vi "General Block Diagram.vi"() -> ()   [LabVIEW 2017]
panel:
  out "Current Forearm\nAngle":dbl
  out "Current Backarm\nAngle":dbl
  in  "Initial Parametric\nValue":dbl format="%#_13g"
  in  "Initial Forearm\nAngle":dbl format="%#_13g"
  in  "Initial Backarm\nAngle":dbl format="%#_13g"
  in  "Forearm Length":dbl format="%#_13g"
  in  "Backarm Length":dbl format="%#_13g"
  in  "New Parametric\nValue":dbl
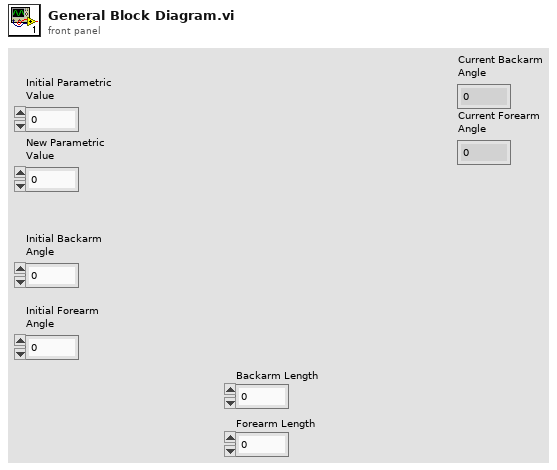
[diagram p1: front panel]
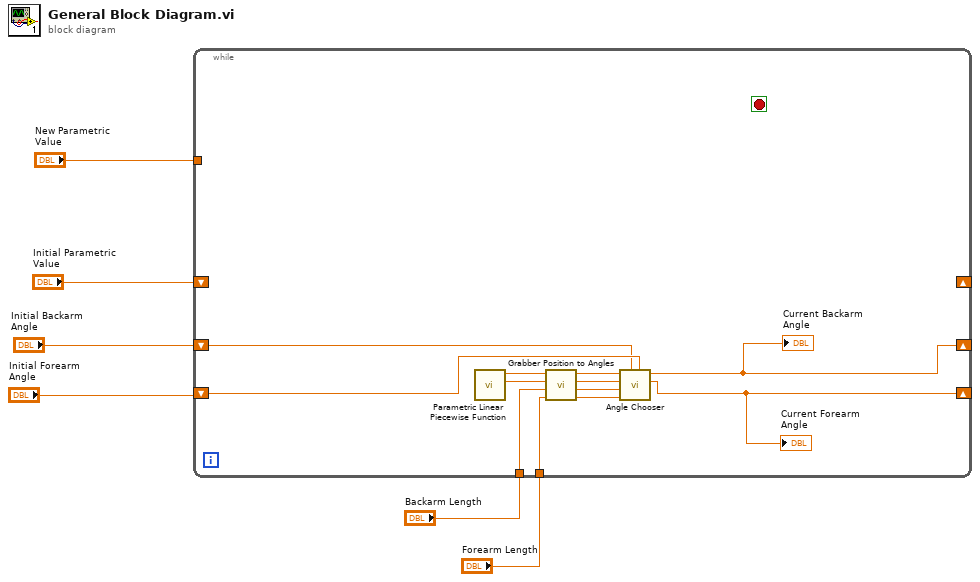
[diagram p0: block diagram]
diagram:
  n1 = while {
    shift-right: _ -> [_]
    shift-left: "Initial Parametric\nValue" -> [_]
    tunnel: "New Parametric\nValue" -> [_]
    tunnel: "Forearm Length" -> [w12]
    tunnel: "Backarm Length" -> [w11]
    shift-right: [w8] -> _
    shift-left: "Initial Backarm\nAngle" -> [w9]
    shift-right: [w7] -> _
    shift-left: "Initial Forearm\nAngle" -> [w10]
    stop <- _ stop-if-true
    n2 = call "Parametric Linear Piecewise Function.vi"() -> ("Y Position"=w17:dbl, "X Position"=w18:dbl)  [unwired: 10 in]
    n3 = call "Grabber Position to Angles.vi"("Forearm Length"=w12, "Backarm Length"=w11, "Y Initial"=w17, "X Initial"=w18) -> ("Forearm Angle\nDegrees 2"=w13:dbl, "Backarm Angle\nDegrees 2"=w14:dbl, "Forearm Angle\nDegrees 1"=w15:dbl, "Backarm Angle\nDegrees 1"=w16:dbl)  [unwired: 4 in]
    n4 = call "Angle Chooser.vi"("Forearm Angle Initial"=w10, "Backarm Angle Initial"=w9, "Forearm Angle 2"=w13, "Backarm Angle 2"=w14, "Forearm Angle 1"=w15, "Backarm Angle 1"=w16) -> ("final Forearm Angle"=w7:dbl, "final Backarm Angle"=w8:dbl)  [unwired: 4 in]
    "Current Backarm\nAngle" <- w8
    "Current Forearm\nAngle" <- w7
  }
